vi "Get Screen Dump.vi"(8 "error in (no error)":errorcluster, 9 "Path (C:\\Users\\Public\\Pictures\\AG3352X)":path=path "C:/Users/Public/Pictures/AG3352X", 10 "Image Format (1: BMP)":i32(ring)=1 items=["PNG", "BMP"], 11 "VISA resource name":refnum<visa-resource-name>) -> (0 "error out":errorcluster, 3 "VISA resource name out":refnum<visa-resource-name>)   [LabVIEW 2019, in "Agilent 3352X Series.lvlib"]
doc: "Captures and save the front-panel display image in specified format to specific local pc path."
uses:
  Agilent 3352X Series.lvlib
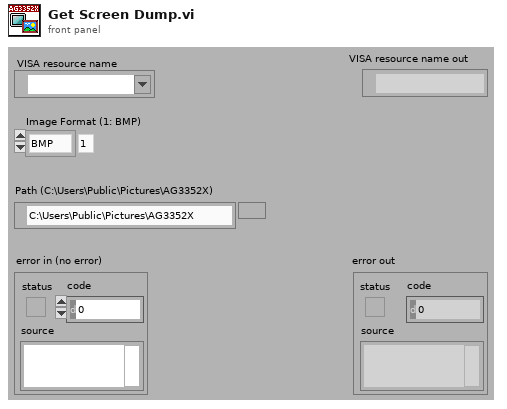
[diagram p1: front panel]
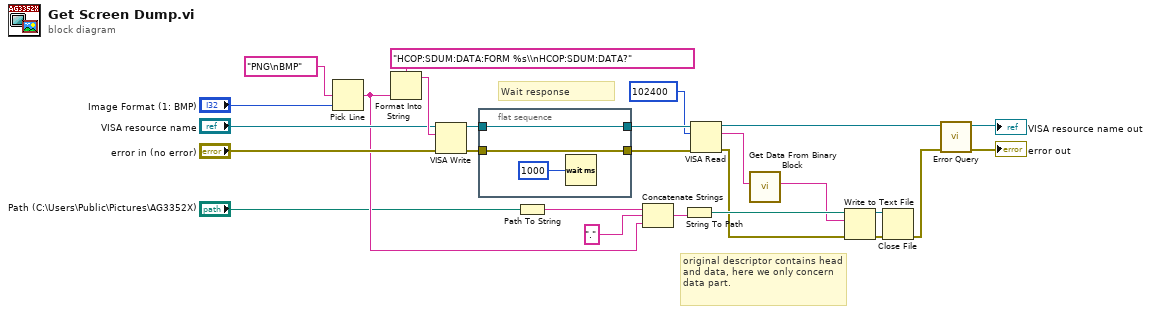
[diagram p0: block diagram]
diagram:
  # "original descriptor contains head and data, here we only concern data part."
  # "Wait response"
  n1 = Pick Line(multi-line string="PNG\nBMP", line index="Image Format (1: BMP)") -> (output string=w17:string)  [unwired: 1 out]
  n2 = Format Into String(format string="HCOP:SDUM:DATA:FORM %s\\nHCOP:SDUM:DATA?", w17) -> (resulting string=w25:string)  [unwired: 2 in, 1 out]
  n3 = VISA Write(VISA resource name="VISA resource name", write buffer=w25, error in (no error)="error in (no error)") -> (VISA resource name out=w20:refnum<visa-resource-name>, error out=w19:errorcluster)  [unwired: 1 out]
  n4 = flat-sequence {
    tunnel: w20 -> [w28]
    tunnel: w19 -> [w27]
    tunnel: [w28] -> w13
    tunnel: [w27] -> w12
    frame #0 {
      n5 = Wait (ms)(milliseconds to wait=u32 1000) -> ()  [unwired: 1 out]
    }
  }
  n6 = Path To String(path="Path (C:\\Users\\Public\\Pictures\\AG3352X)") -> (string=w18:string)
  n7 = Concatenate Strings(w18, "." ("string"), w17) -> (w14:string)
  n8 = String To Path(string=w14) -> (path=w10:path)
  n9 = VISA Read(VISA resource name=w13, byte count=u32 102400, error in (no error)=w12) -> (VISA resource name out=w4:refnum<visa-resource-name>, read buffer=w9:string, error out=w7:errorcluster)  [unwired: 1 out]
  n10 = call "Get Data From Binary Block.vi"("Binary Block"=w9) -> ("Data Part"=w8:string)  [unwired: 10 out]
  n11 = Write to Text File(file (use dialog)=w10, text=w8, error in=w7) -> (refnum out=w6:refnum<file>, error out=w5:errorcluster)  [unwired: 2 out]
  n12 = Close File(refnum=w6, error in=w5) -> (error out=w2:errorcluster)  [unwired: 1 out]
  n13 = call "Error Query.vi"("error in (no error)"=w2, "VISA resource name"=w4) -> ("error out"=→"error out":errorcluster, "VISA resource name out"=→"VISA resource name out":refnum<visa-resource-name>)  [unwired: 8 out]
